vi "Reset DAQmx.vi"(8 "error in (no error)":errorcluster) -> (0 "error out":errorcluster)   [LabVIEW 2019, in "Reset Hardware Engine.lvlib"]
uses:
  Reset Hardware Engine.lvlib
  <vilib>/nisyscfg/Close (Hardware).vi
  <vilib>/nisyscfg/Close (Filter).vi
  <vilib>/nisyscfg/Close (System).vi
  <resource>/objmgr/nicontrollersysapi.rc
  <vilib>/nisyscfg/nisyscfg.lvlib
  <vilib>/NI VeriStand/Custom Device Tools/Custom Device Utility Library/Custom Device Utility Library.lvlib
  <resource>/objmgr/niflexrioatomicsae.rc
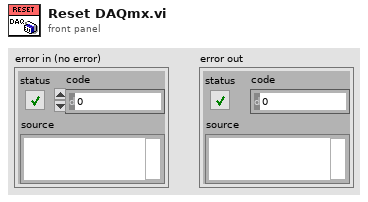
[diagram p1: front panel]
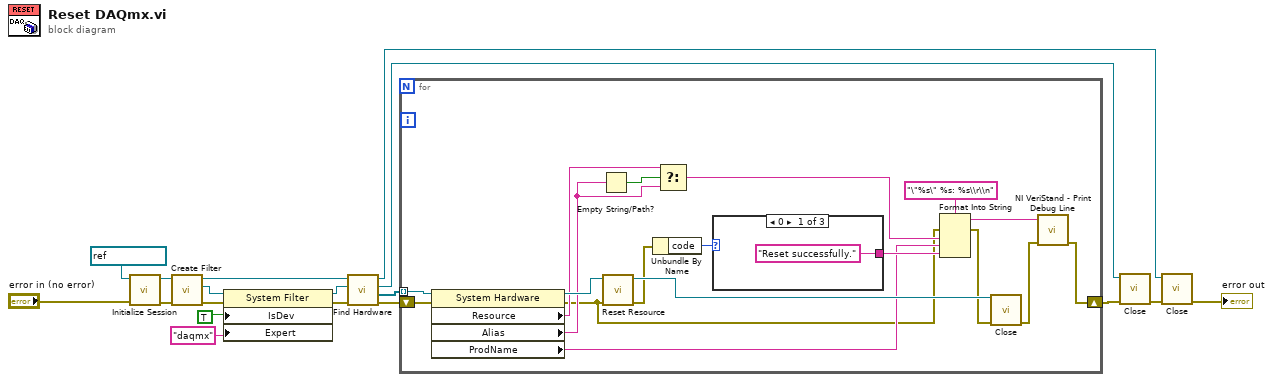
[diagram p0: block diagram]
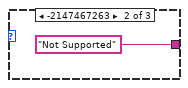
[diagram p2: hidden frame]
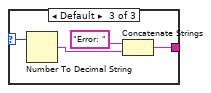
[diagram p3: hidden frame]
diagram:
  n1 = call <vilib>:"Initialize Session.vi"("error in (no error)"="error in (no error)", "Target (localhost)"=refnum<k21> "localhost") -> ("error out"=w5:errorcluster, "Session out"=w4:refnum<k21>)  [unwired: 8 in]
  n2 = call <vilib>:"Create Filter.vi"("error in (no error)"=w5, "Session in"=w4) -> ("error out"=w9:errorcluster, "Filter out"=w6:refnum<k20>, "Session out"=w3:refnum<k21>)  [unwired: 7 in]
  n3 = property class="System Filter"(reference=w6, error in=w9, "IsDev"=TRUE ("Is Device"), "Expert"="daqmx" ("Expert Info:Expert Name")) -> (reference out=w7:refnum<k20>, error out=w10:errorcluster)
  n4 = call <vilib>:"Find Hardware.vi"("error in (no error)"=w10, "Filter in"=w7, "Session in"=w3) -> ("error out"=w2:errorcluster, "Resources out"=w1:refnum<k20>[], "Filter out"=w13:refnum<k20>, "Session out"=w14:refnum<k21>)  [unwired: 1 in, 4 out]
  n5 = for {
    tunnel: w1 -> [w35] mode=indexing
    shift-right: [w20] -> w12
    shift-left: w2 -> [w34]
    n6 = property class="System Hardware"(reference=w35, error in=w34) -> (reference out=w33:refnum<k20>, error out=w23:errorcluster, "Resource"=w29:string, "Alias"=w28:string, "ProdName"=w25:string)
    n7 = Empty String/Path?(string/path=w28) -> (empty?=w36:bool)
    n8 = call <vilib>:"Reset Resource.vi"("error in (no error)"=w23, "Resource in"=w33) -> ("error out"=w30:errorcluster, "Resource out"=w32:refnum<k20>)  [unwired: 6 in, 2 out]
    n9 = Unbundle By Name(w30) -> ("code"=w31:i32)
    n10 = Select(t=w29, s=w36, f=w28) -> (s? t:f=w24:string)
    n11 = case shown="0" w31 {
      selector: w31 -> [_ _ w40]
      tunnel: ["Reset successfully." ("L10n_Pass") "Not Supported" ("L10n_NotSupported") w39] -> w26
      frame 0 {
      }
      frame -2147467263 {
      }
      frame Default {
        n12 = Number To Decimal String(number=w40) -> (decimal integer string=w42:string)  [unwired: 1 in]
        n13 = Concatenate Strings("Error: " ("L10n_Error"), w42) -> (w39:string)
      }
    }
    n14 = Format Into String(format string="\"%s\" %s: %s\\r\\n", error in=w23, w24, w25, w26) -> (resulting string=w19:string, error out=w22:errorcluster)  [unwired: 1 in]
    n15 = call-poly <vilib>:"Close.vi"("error in (no error)"=w22, "Resource in"=w32) -> ("error out"=w21:errorcluster)  [unwired: 9 in]
    n16 = call <vilib>:"NI VeriStand - Print Debug Line.vi"("error in (no error)"=w21, "Message"=w19) -> ("error out"=w20:errorcluster)  [unwired: 9 in]
  }
  n17 = call-poly <vilib>:"Close.vi"("error in (no error)"=w12, "Filter in"=w13) -> ("error out"=w11:errorcluster)  [unwired: 9 in]
  n18 = call-poly <vilib>:"Close.vi"("error in (no error)"=w11, "Session in"=w14) -> ("error out"=→"error out":errorcluster)  [unwired: 9 in]
